vi "ADS Type Byte Stream to Variant.vi"(7 "Type Name":string, 8 "error in (no error)":errorcluster, 10 "Byte Stream":u8[](array[numeric]), 11 "TwinCAT ADS in":refnum<class "TwinCAT ADS.lvclass">) -> (0 "error out":errorcluster, 2 "Value":variant, 3 "TwinCAT ADS out":refnum<class "TwinCAT ADS.lvclass">)   [LabVIEW 2018, in "TwinCAT ADS.lvclass"]
uses:
  TwinCAT ADS.lvclass
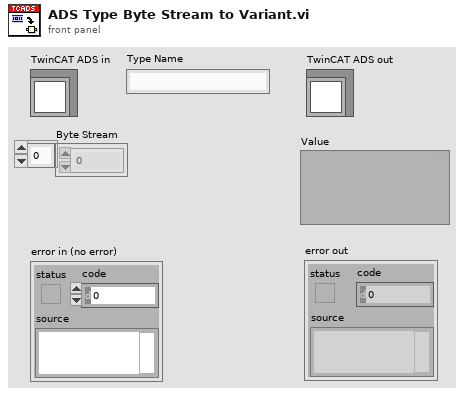
[diagram p1: front panel]
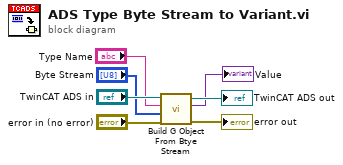
[diagram p0: block diagram]
diagram:
  n1 = call "Build G Object From Btye Stream.vi"("error in (no error)"="error in (no error)", "Byte Stream in"="Byte Stream", "Type Name"="Type Name", "TwinCAT ADS in"="TwinCAT ADS in") -> ("error out"=→"error out":errorcluster, "Value"=→"Value":variant, "TwinCAT ADS out"=→"TwinCAT ADS out":refnum<class "TwinCAT ADS.lvclass">)  [unwired: 4 in, 1 out]
